vi "ESA-C GPIB Selector.vi"(1 "Drive Connection Settings":T1={"Objective GPIB-Port"=4, "Stage GPIB-Port"=4, "Drive Selector"=0, "Drive Velocity (V/s)"=5.0} {"Drive Velocity (V/s)" min=10.0 max=160.0 step=0.1 format="%.1f"; "Drive Selector" items=["Obj.", "Stage"]; "Stage GPIB-Port" min=1 max=20 step=1 format="%#.0f"; "Objective GPIB-Port" min=1 max=20 step=1 format="%#.0f"}) -> (0 "String":string)   [LabVIEW 2010]
uses:
  TypeDefs/ESA-C Connection Settings.ctl
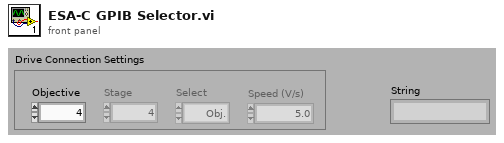
[diagram p1: front panel]
types:
  T1 = typedef "ESA-C Connection Settings.ctl" = cluster{"Objective GPIB-Port":i32, "Stage GPIB-Port":i32, "Drive Selector":u16, "Drive Velocity (V/s)":dbl}
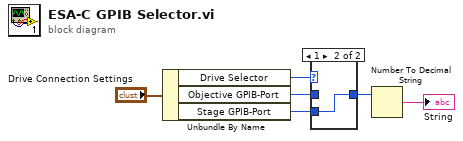
[diagram p0: block diagram]
diagram:
  n1 = Unbundle By Name("Drive Connection Settings") -> ("Drive Selector"=w4:u16, "Objective GPIB-Port"=w6:i32, "Stage GPIB-Port"=w5:i32)
  n2 = case shown="1" w4 {
    tunnel: [w7 w8] -> w3
    tunnel: w5 -> [_ w8]
    tunnel: w6 -> [w7 _]
    frame 0, Default {
    }
    frame 1 {
    }
  }
  n3 = Number To Decimal String(number=w3) -> (decimal integer string=→"String":string)  [unwired: 1 in]
